vi "homework - display CSV data.vi"() -> ()   [LabVIEW 2024]
doc: "#vi_description \nOpens a CSV file and displays the data on screen.\nThetic Engineering Ltd."
uses:
  <vilib>/Utility/file.llb/Read Delimited Spreadsheet (string).vi
panel:
  in  "Path to CSV":path
  out "Table of Data":string[][](table)
  out "Graph of Data":dbl[][](graph)
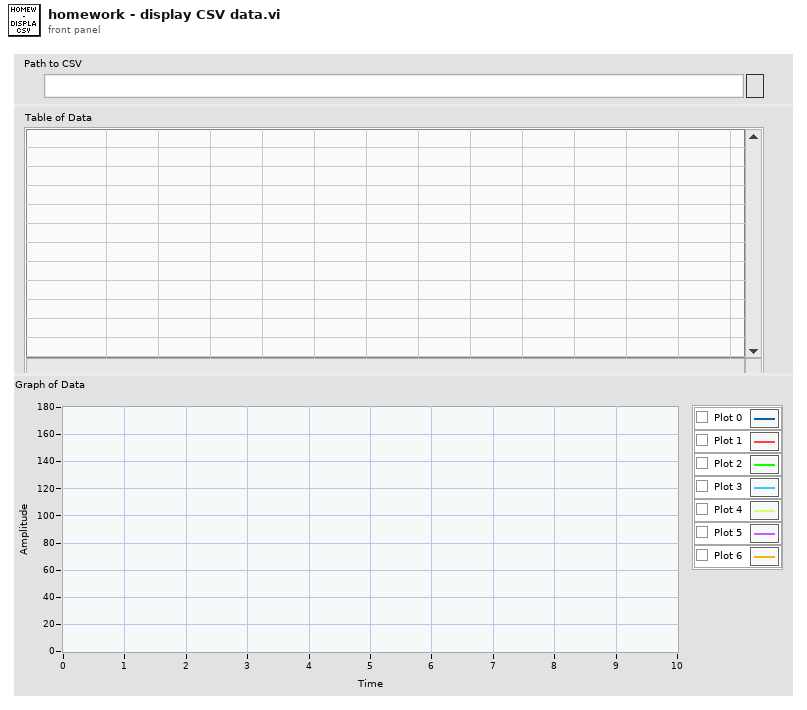
[diagram p1: front panel]
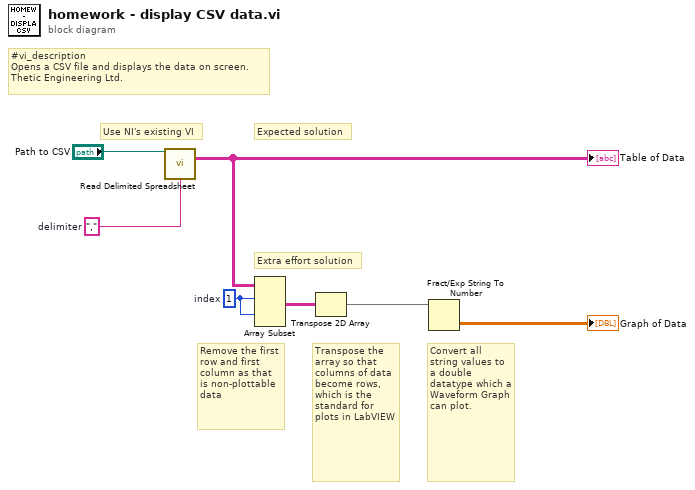
[diagram p0: block diagram]
diagram:
  w4 = 1  # index
  w6 = ","  # delimiter
  # "Convert all string values to a double datatype which a Waveform Graph can plot."
  # "Transpose the array so that columns of data become rows, which is the standard for plots in LabVIEW"
  # "Remove the first row and first column as that is non-plottable data"
  # "Use NI's existing VI"
  # "Extra effort solution"
  # "Expected solution"
  # "#vi_description \nOpens a CSV file and displays the data on screen.\nThetic Engineering Ltd."
  n1 = call-poly <vilib>:"Read Delimited Spreadsheet.vi"("file path (dialog if empty)"="Path to CSV", "delimiter (\\t)"=w6) -> ("all rows"=w5:string[][])  [unwired: 8 in, 5 out]
  "Table of Data" <- w5
  n2 = Array Subset(array=w5, index (row)=w4, index (col)=w4) -> (w3:string[][])  [unwired: 2 in]
  n3 = Transpose 2D Array(2D array=w3) -> (transposed array=w2:string[][])
  n4 = Fract/Exp String To Number(string=w2) -> (number=→"Graph of Data":dbl[][])  [unwired: 3 in, 1 out]
